vi "Paskevits_Vladislav_kt1.vi"() -> ()   [LabVIEW 2018]
doc: "This vi will read text file and write two type of data in to different text files.\nExtract values and show them on different graphs."
panel:
  out "remaining string":string
  out "appended array":dbl[](array[numeric])
  out "Waveform Chart":dbl(graph)
  out "Waveform Graph":dbl[](graph)
  out "substring":string
  in  "Stop":bool
  out "Input":string
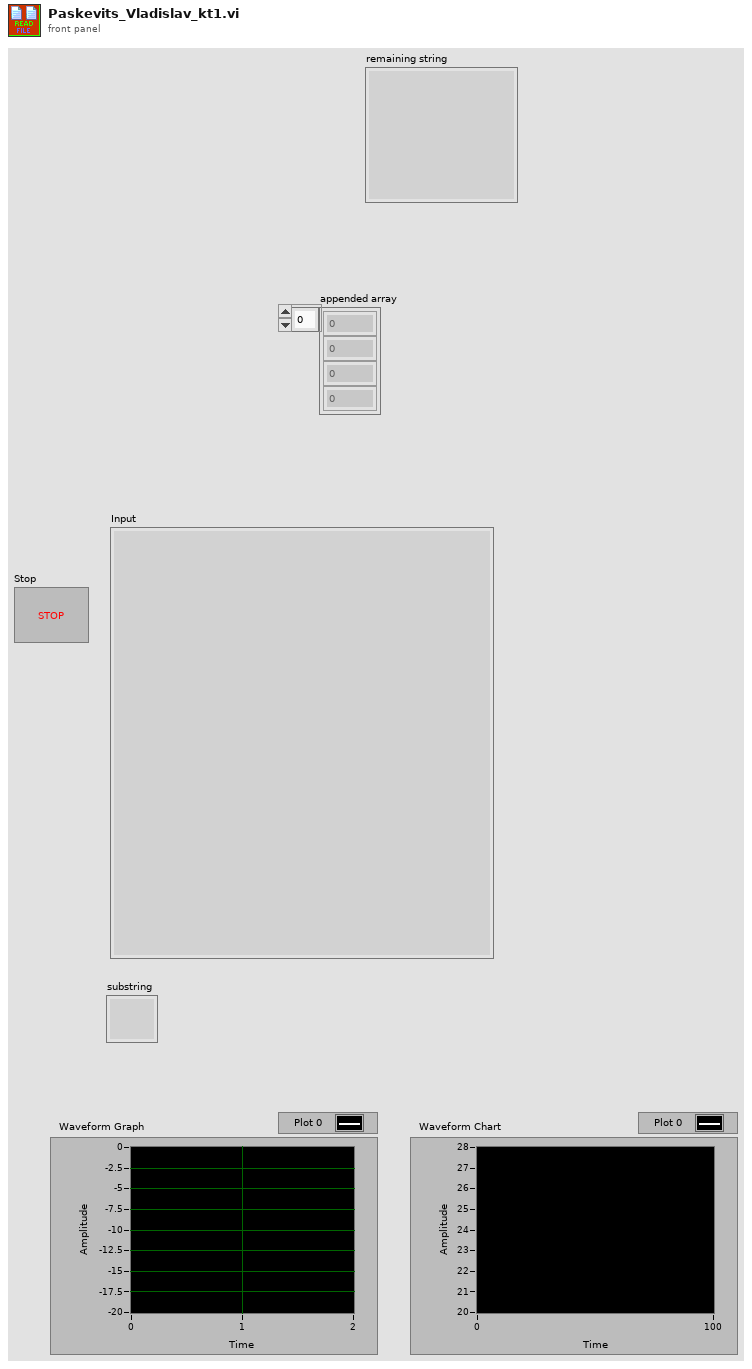
[diagram p1: front panel]
types:
  T1 = enum16{"open", "replace", "create", "open or create", "replace or create", "replace or create with confirmation"}
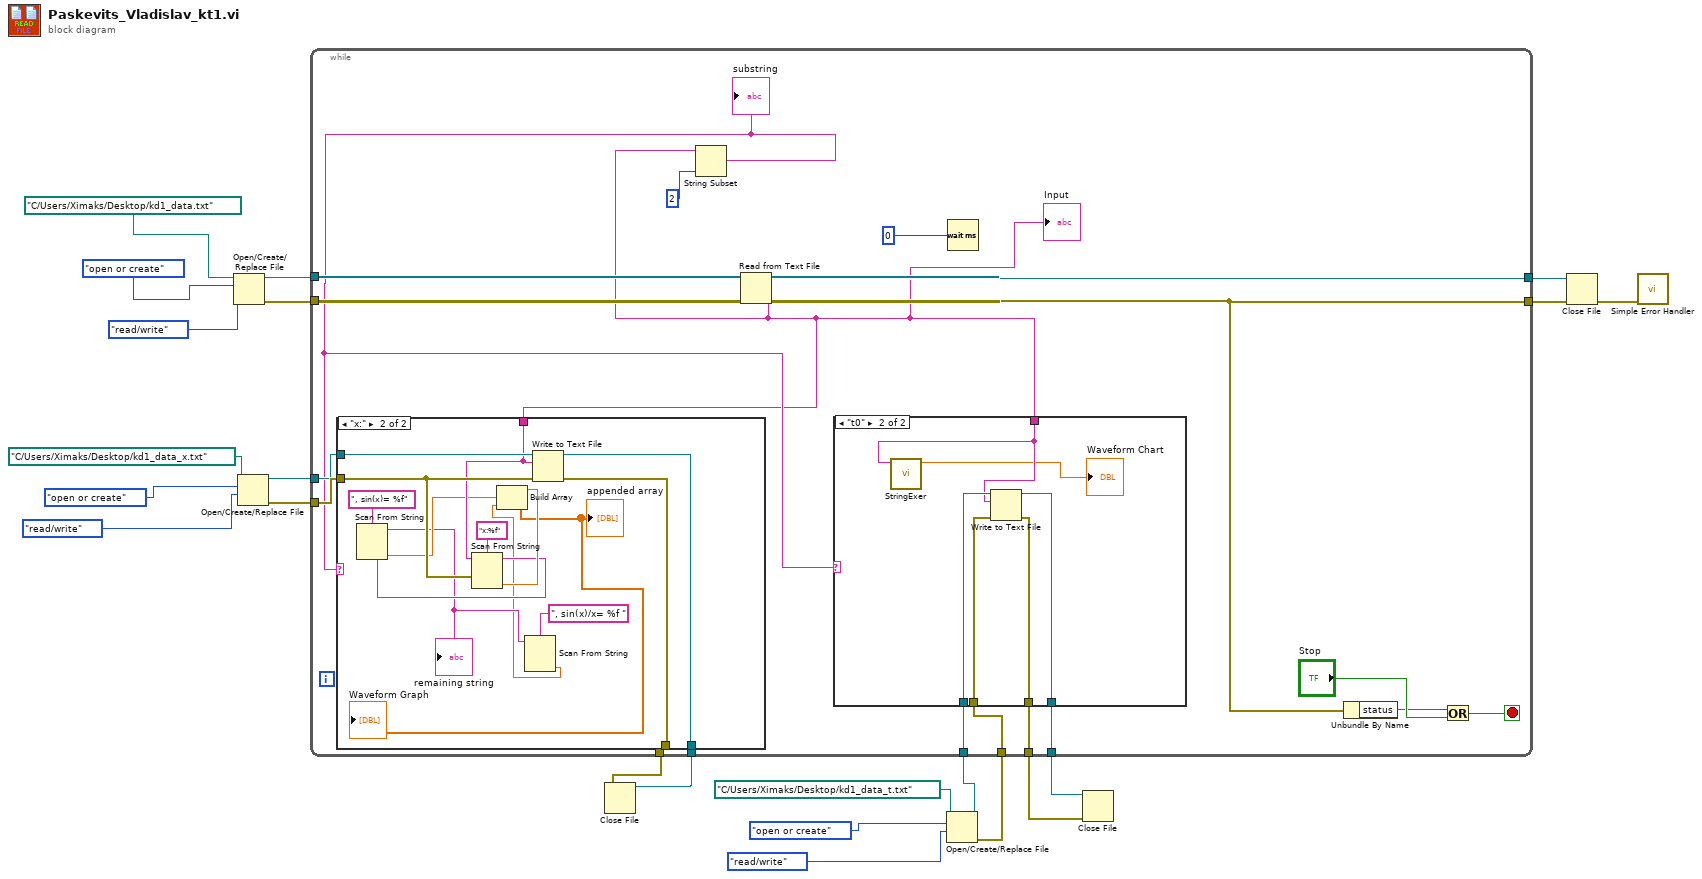
[diagram p0: block diagram]
diagram:
  n1 = Open/Create/Replace File(file path (use dialog)=path "C:/Users/Ximaks/Desktop/kd1_data.txt", operation (0:open)=T1."open or create", access (0:read/write)=enum16{"read/write", "read-only", "write-only"}."read/write") -> (refnum out=w22:refnum<file>, error out=w15:errorcluster)  [unwired: 3 in, 1 out]
  n2 = Open/Create/Replace File(file path (use dialog)=path "C:/Users/Ximaks/Desktop/kd1_data_x.txt", operation (0:open)=T1."open or create", access (0:read/write)=enum16{"read/write", "read-only", "write-only"}."read/write") -> (refnum out=w5:refnum<file>, error out=w6:errorcluster)  [unwired: 3 in, 1 out]
  n3 = Open/Create/Replace File(file path (use dialog)=path "C:/Users/Ximaks/Desktop/kd1_data_t.txt", operation (0:open)=T1."open or create", access (0:read/write)=enum16{"read/write", "read-only", "write-only"}."read/write") -> (refnum out=w10:refnum<file>, error out=w11:errorcluster)  [unwired: 3 in, 1 out]
  n4 = while {
    tunnel: w22 -> [w35]
    tunnel: w15 -> [w34]
    tunnel: [w36] -> w19
    tunnel: [w37] -> w18
    tunnel: w11 -> [w33]
    tunnel: w10 -> [w32]
    tunnel: w6 -> [w31]
    tunnel: w5 -> [w30]
    tunnel: [w29] -> w4
    tunnel: [w28] -> w3
    tunnel: [w26] -> w2
    tunnel: [w25] -> w1
    stop <- w40 stop-if-true
    n5 = Read from Text File(file (use dialog)=w35, error in=w34) -> (refnum out=w36:refnum<file>, text=w23:string, error out=w37:errorcluster)  [unwired: 2 in, 1 out]
    "Input" <- w23
    n6 = String Subset(string=w23, length (rest)=2 ("length (rest)")) -> (substring=w24:string)  [unwired: 1 in]
    "substring" <- w24
    n7 = case shown="\"x:\"" w24 {
      tunnel: w31 -> [w50 w61]
      tunnel: w30 -> [w51 w65]
      tunnel: [w50 w64] -> w29
      tunnel: [w51 w63] -> w28
      tunnel: w23 -> [_ w59]
      frame "", Default {
      }
      frame "x:" {
        n8 = Scan From String(format string="x:%f", input string=w59, error in=w61) -> (remaining string=w57:string, output 1=w60:dbl)  [unwired: 2 in, 2 out]
        n9 = Scan From String(format string=", sin(x)= %f", input string=w57) -> (remaining string=w54:string, output 1=w55:dbl)  [unwired: 3 in, 2 out]
        "remaining string" <- w54
        n10 = Scan From String(format string=", sin(x)/x= %f ", input string=w54) -> (output 1=w52:dbl)  [unwired: 3 in, 3 out]
        n11 = Build Array(w60, w55, w52) -> (→"appended array" →"Waveform Graph":dbl[])
        n12 = Write to Text File(file (use dialog)=w65, text=w59, error in=w61) -> (refnum out=w63:refnum<file>, error out=w64:errorcluster)  [unwired: 1 in, 1 out]
      }
    }
    n13 = case shown="\"t0\"" w24 {
      tunnel: w33 -> [w43 w49]
      tunnel: w32 -> [w42 w48]
      tunnel: [w42 w47] -> w26
      tunnel: [w43 w46] -> w25
      tunnel: w23 -> [_ w45]
      frame "", Default {
      }
      frame "t0" {
        n14 = call "StringExer.vi"("String"=w45) -> ("Temperature"=→"Waveform Chart":dbl)  [unwired: 9 in, 1 out]
        n15 = Write to Text File(file (use dialog)=w48, text=w45, error in=w49) -> (refnum out=w47:refnum<file>, error out=w46:errorcluster)  [unwired: 1 in, 1 out]
      }
    }
    n16 = Wait (ms)(milliseconds to wait=0) -> ()  [unwired: 1 out]
    n17 = Unbundle By Name(w37) -> ("status"=w38:bool)
    n18 = Or(x=w38, y="Stop") -> (x .or. y?=w40:bool)
  }
  n19 = Close File(refnum=w3, error in=w4) -> ()  [unwired: 2 out]
  n20 = Close File(refnum=w2, error in=w1) -> ()  [unwired: 2 out]
  n21 = Close File(refnum=w19, error in=w18) -> (error out=w17:errorcluster)  [unwired: 1 out]
  n22 = call <vilib>:"Simple Error Handler.vi"("error in (no error)"=w17) -> ()  [unwired: 4 in, 5 out]
